vi "Board Write to File.vi"(8 "error in (no error)":errorcluster, 10 "Path":path, 11 "Board in":refnum<class "Board.lvclass">) -> (0 "error out":errorcluster, 3 "Board out":refnum<class "Board.lvclass">)   [LabVIEW 2019, in "Board.lvclass"]
uses:
  Board.lvclass
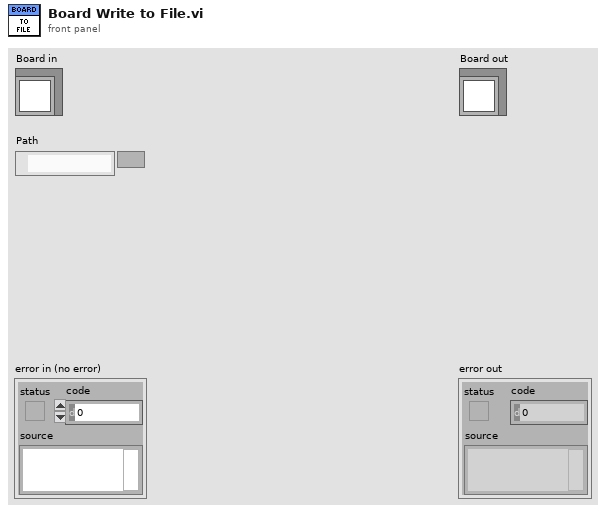
[diagram p1: front panel]
types:
  T1 = enum16{"open", "replace", "create", "open or create", "replace or create", "replace or create with confirmation"}
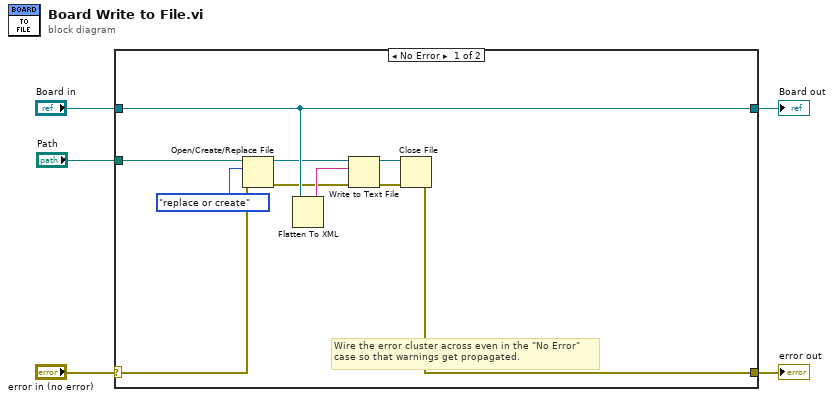
[diagram p0: block diagram]
diagram:
  n1 = case shown="No Error" "error in (no error)" {
    selector: "error in (no error)" -> [w7 w17]
    tunnel: [w6 w17] -> w4
    tunnel: [w13 w16] -> w2
    tunnel: "Board in" -> [w13 w16]
    tunnel: "Path" -> [w15 _]
    frame No Error {
      # "Wire the error cluster across even in the \"No Error\"\ncase so that warnings get propagated."
      n2 = Open/Create/Replace File(file path (use dialog)=w15, error in=w7, operation (0:open)=T1."replace or create") -> (refnum out=w12:refnum<file>, error out=w10:errorcluster)  [unwired: 3 in, 1 out]
      n3 = Flatten To XML(anything=w13) -> (xml string=w11:string)
      n4 = Write to Text File(file (use dialog)=w12, text=w11, error in=w10) -> (refnum out=w8:refnum<file>, error out=w9:errorcluster)  [unwired: 1 in, 1 out]
      n5 = Close File(refnum=w8, error in=w9) -> (error out=w6:errorcluster)  [unwired: 1 out]
    }
    frame Error {
    }
  }
  "error out" <- w4
  "Board out" <- w2
